vi "DOE Channel Test Labels.vi"(0 "RunTime":bool) -> (4 "Agilent Cluster Array":T2[](array[typedef]), 6 "Channel List":string)   [LabVIEW 2013]
uses:
  Type Definitions/Channel Label.ctl
  Type Definitions/Agilent Cluster.ctl
  <vilib>/Utility/file.llb/Write To Spreadsheet File (string).vi
  <vilib>/Utility/file.llb/Read From Spreadsheet File (string).vi
panel:
  in  "Sensor 5":T1
  in  "Read TC Tree":bool
  out "Description":string="DAQ Setup"
  in  "Tab Control":enum32{"Page 1", "Page 2"}(tab)
  out "Agilent TC Locations":string[][](array[string])
  in  "Read":bool
  in  "Write":bool
  in  "Sensor 4":T1
  in  "Read None":bool
  in  "Sensor 3":T1
  in  "Read All":bool
  in  "Complete":bool
  in  "Panel 3":T1[][](array[typedef])=[[{"Label"="TC Cond1 - IN", "Chan"="301", "Rec"=TRUE, "Unit"=""}, {"Label"="TC Cond2", "Chan"="302", "Rec"=TRUE, "Unit"=""}, {"Label"="TC Cond3", "Chan"="303", "Rec"=TRUE, "Unit"=""}, {"Label"="TC Cond4", "Chan"="304", "Rec"=TRUE, "Unit"=""}, {"Label"="TC Cond5", "Chan"="305", "Rec"=TRUE, "Unit"=""}, {"Label"="TC Cond6", "Chan"="306", "Rec"=TRUE, "Unit"=""}], [{"Label"="TC Cond7", "Chan"="307", "Rec"=TRUE, "Unit"=""}, {"Label"="TC Cond8", "Chan"="308", "Rec"=TRUE, "Unit"=""}, {"Label"="TC Cond9", "Chan"="309", "Rec"=TRUE, "Unit"=""}, {"Label"="TC Cond10", "Chan"="310", "Rec"=TRUE, "Unit"=""}, {"Label"="TC Cond11", "Chan"="311", "Rec"=TRUE, "Unit"=""}, {"Label"="TC Cond12 - OUT", "Chan"="312", "Rec"=TRUE, "Unit"=""}], [{"Label"="TC Xtra 4", "Chan"="313", "Rec"=TRUE, "Unit"=""}, {"Label"="TC Xtra 5", "Chan"="314", "Rec"=TRUE, "Unit"=""}, {"Label"="TC Xtra 6", "Chan"="315", "Rec"=TRUE, "Unit"=""}, {"Label"="TC Xtra 7", "Chan"="316", "Rec"=TRUE, "Unit"=""}, {"Label"="TC Xtra 8", "Chan"="105", "Rec"=TRUE, "Unit"=""}, {"Label"="TC Xtra 9", "Chan"="106", "Rec"=TRUE, "Unit"=""}]]
  in  "Panel 2":T1[][](array[typedef])=[[{"Label"="TC Dry/W bulb 1", "Chan"="201", "Rec"=TRUE, "Unit"=""}, {"Label"="TC Dry/W bulb 2", "Chan"="202", "Rec"=TRUE, "Unit"=""}, {"Label"="TC Dry/W bulb 3", "Chan"="203", "Rec"=TRUE, "Unit"=""}, {"Label"="TC Dry/W bulb 4", "Chan"="204", "Rec"=TRUE, "Unit"=""}, {"Label"="TC Tsuction", "Chan"="205", "Rec"=TRUE, "Unit"=""}, {"Label"="TC Tdis", "Chan"="206", "Rec"=TRUE, "Unit"=""}], [{"Label"="TC Tret", "Chan"="207", "Rec"=TRUE, "Unit"=""}, {"Label"="TC Controls 1", "Chan"="208", "Rec"=TRUE, "Unit"=""}, {"Label"="TC Controls 2", "Chan"="209", "Rec"=TRUE, "Unit"=""}, {"Label"="TC Controls 3", "Chan"="210", "Rec"=TRUE, "Unit"=""}, {"Label"="TC Controls 4", "Chan"="211", "Rec"=TRUE, "Unit"=""}, {"Label"="TC Controls 5", "Chan"="212", "Rec"=TRUE, "Unit"=""}], [{"Label"="TC Shadow T1", "Chan"="213", "Rec"=TRUE, "Unit"=""}, {"Label"="TC Shadow T2", "Chan"="214", "Rec"=TRUE, "Unit"=""}, {"Label"="TC Shadow T3", "Chan"="215", "Rec"=TRUE, "Unit"=""}, {"Label"="TC Shadow T4", "Chan"="216", "Rec"=TRUE, "Unit"=""}, {"Label"="TC Shadow T5", "Chan"="107", "Rec"=TRUE, "Unit"=""}, {"Label"="TC Shadow T6", "Chan"="108", "Rec"=TRUE, "Unit"=""}]]
  in  "Panel 1":T1[][](array[typedef])=[[{"Label"="TC Tree 1 - TOP", "Chan"="", "Rec"=TRUE, "Unit"=""}, {"Label"="TC Tree 2", "Chan"="", "Rec"=TRUE, "Unit"=""}, {"Label"="TC Tree 3", "Chan"="", "Rec"=TRUE, "Unit"=""}, {"Label"="TC Tree 4", "Chan"="", "Rec"=TRUE, "Unit"=""}, {"Label"="TC Tree 5", "Chan"="", "Rec"=TRUE, "Unit"=""}, {"Label"="TC Tree 6 - BOT", "Chan"="", "Rec"=TRUE, "Unit"=""}], [{"Label"="TC Shell 1", "Chan"="", "Rec"=TRUE, "Unit"=""}, {"Label"="TC Shell 2", "Chan"="", "Rec"=TRUE, "Unit"=""}, {"Label"="TC Shell 3", "Chan"="", "Rec"=TRUE, "Unit"=""}, {"Label"="TC Shell 4", "Chan"="", "Rec"=TRUE, "Unit"=""}, {"Label"="TC Evap1 - IN", "Chan"="111", "Rec"=TRUE, "Unit"=""}, {"Label"="TC Evap2", "Chan"="112", "Rec"=TRUE, "Unit"=""}], [{"Label"="TC Evap3", "Chan"="113", "Rec"=TRUE, "Unit"=""}, {"Label"="TC Evap4", "Chan"="114", "Rec"=TRUE, "Unit"=""}, {"Label"="TC Evap5 - OUT", "Chan"="115", "Rec"=TRUE, "Unit"=""}, {"Label"="TC Xtra 1", "Chan"="116", "Rec"=TRUE, "Unit"=""}, {"Label"="TC Xtra 2", "Chan"="109", "Rec"=TRUE, "Unit"=""}, {"Label"="TC Xtra 3", "Chan"="1100", "Rec"=TRUE, "Unit"=""}]]
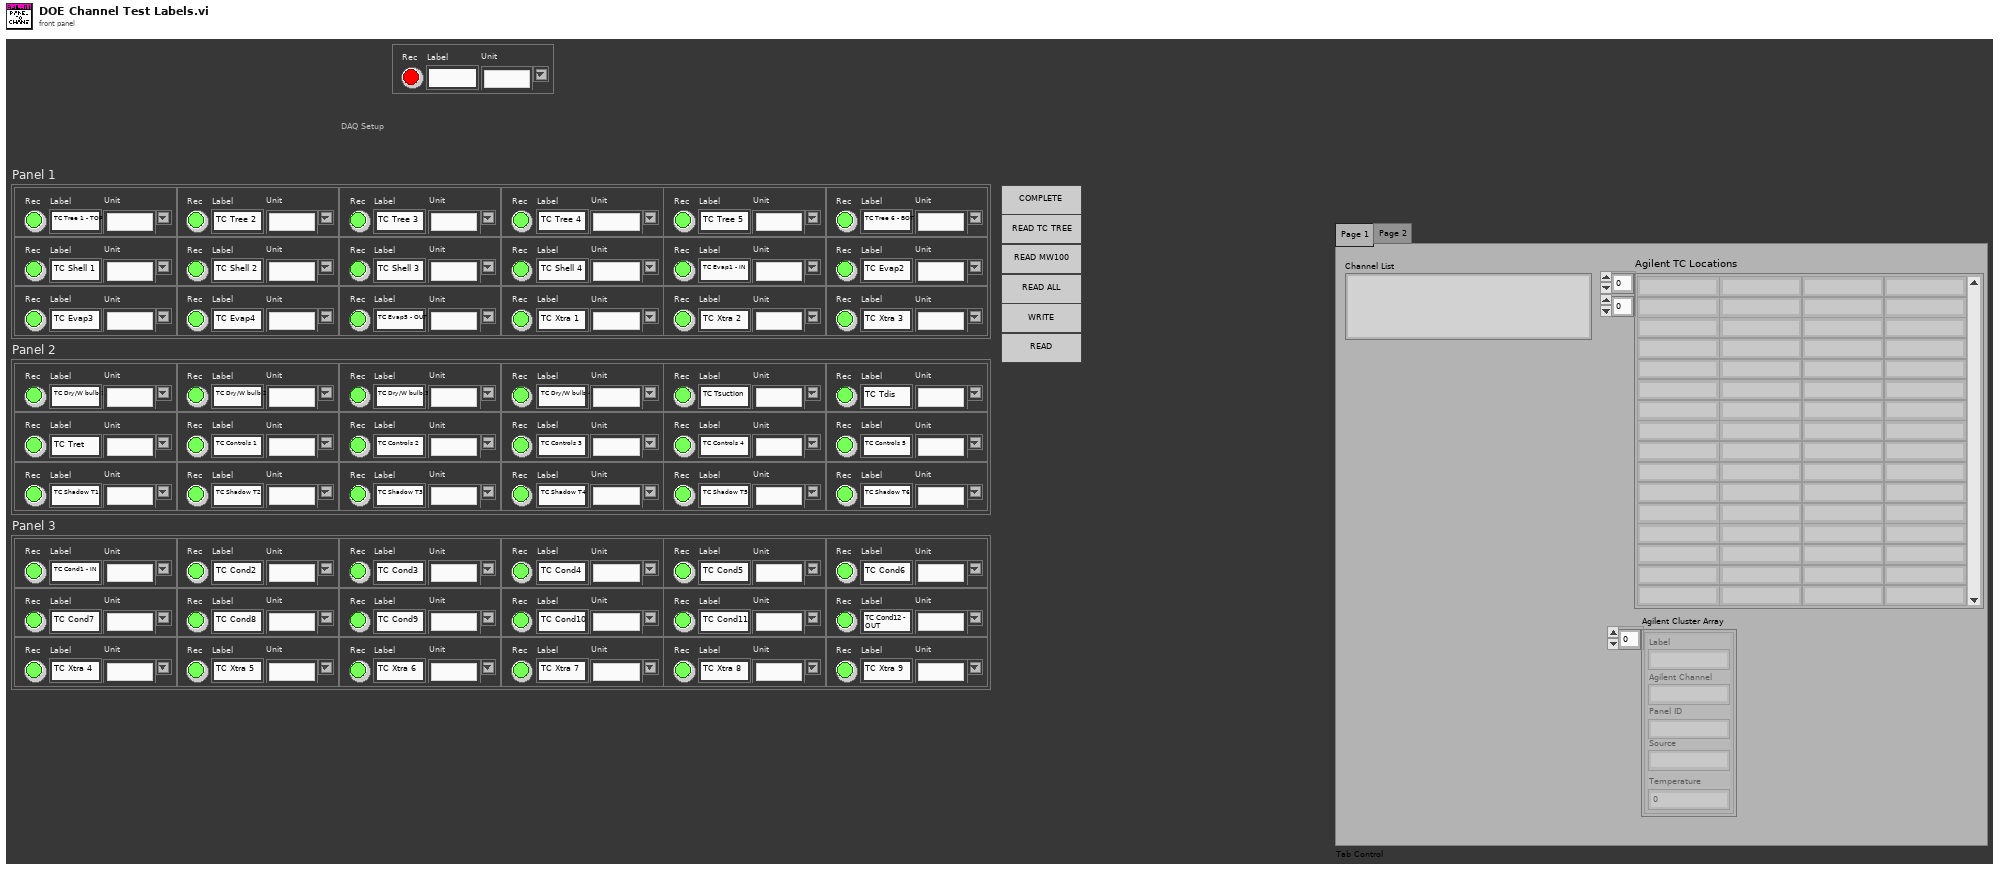
[diagram p1: front panel]
types:
  T1 = typedef "Channel Label.ctl" = cluster{"Label":string, "Chan":string, "Rec":bool, "Unit":string}
  T2 = typedef "Agilent Cluster.ctl" = cluster{"Label":string, "Agilent Channel":string, "Panel ID":string, "Source":string, "Temperature":dbl}
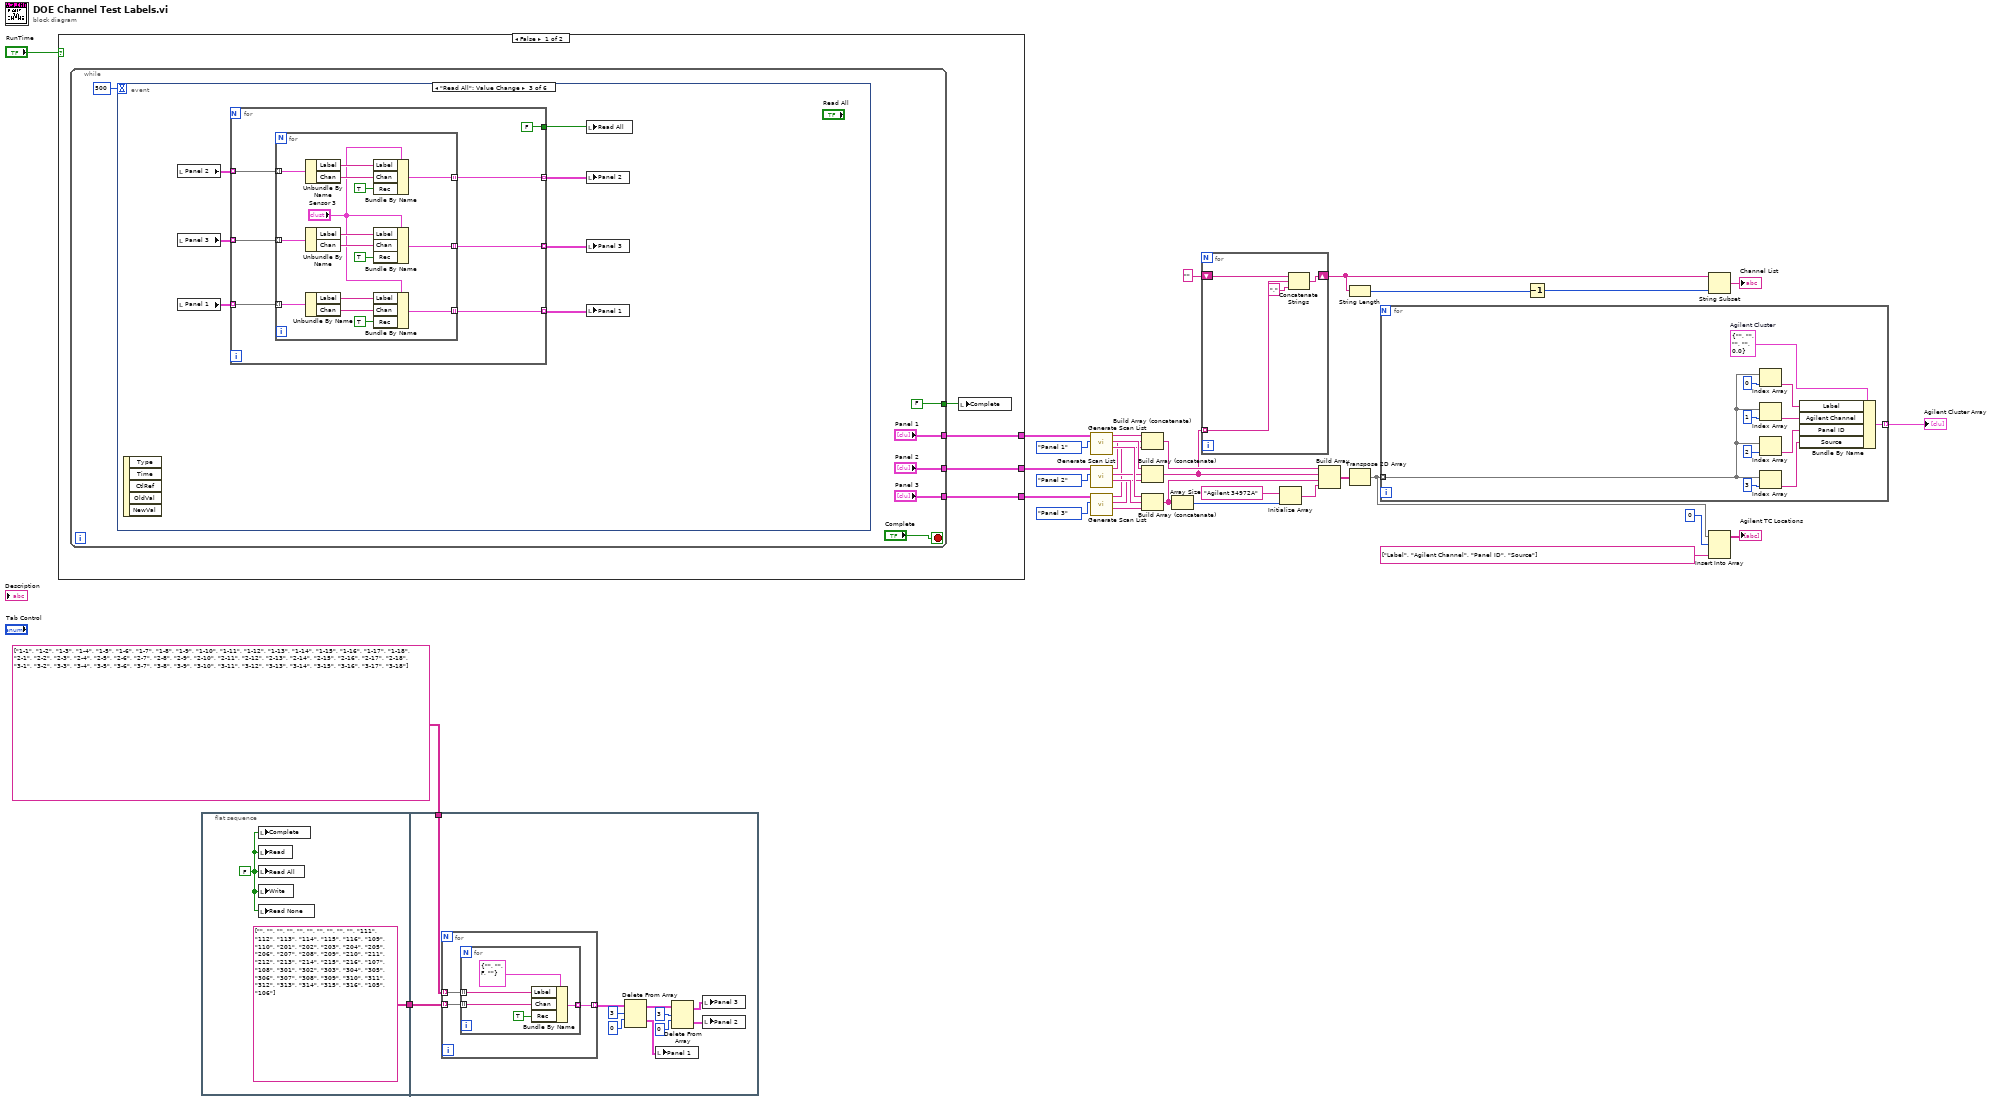
[diagram p0: block diagram]
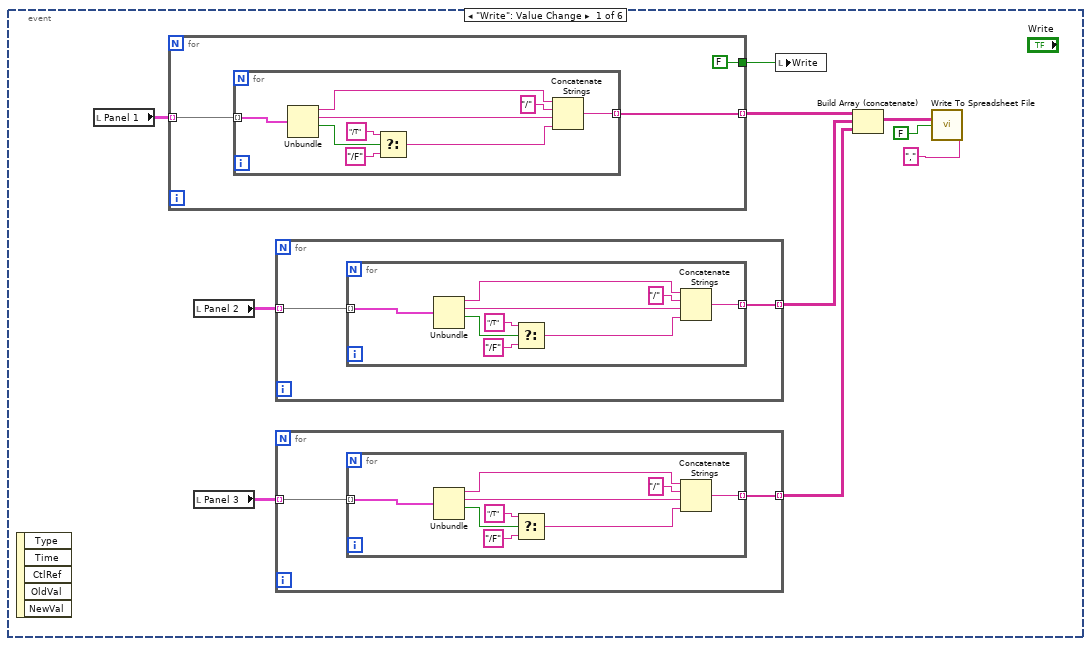
[diagram p2: hidden frame]
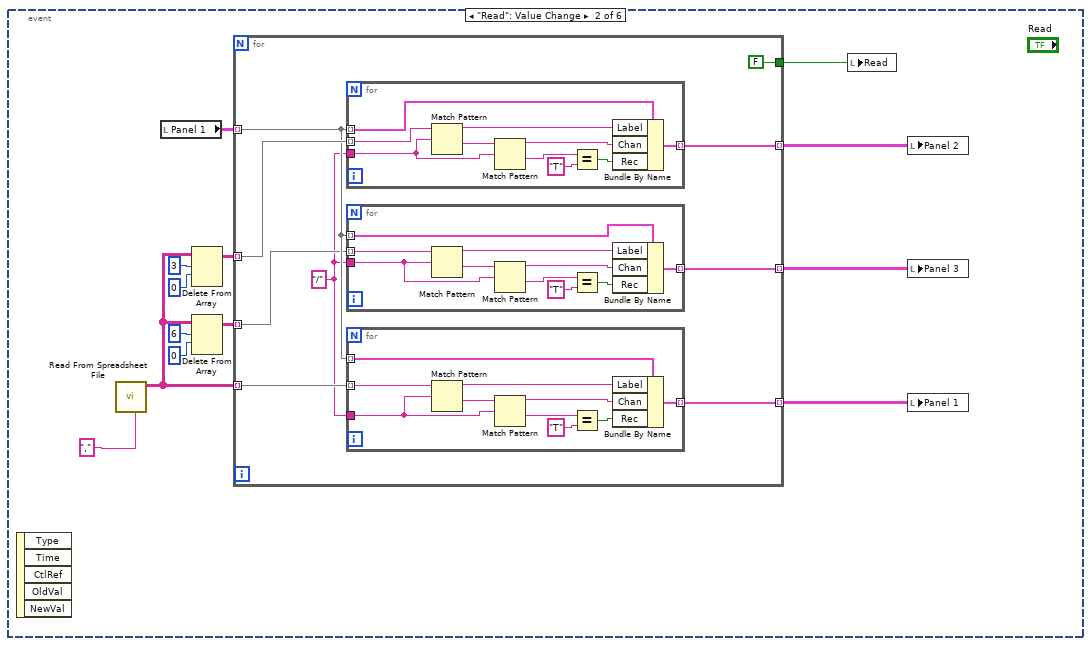
[diagram p3: hidden frame]
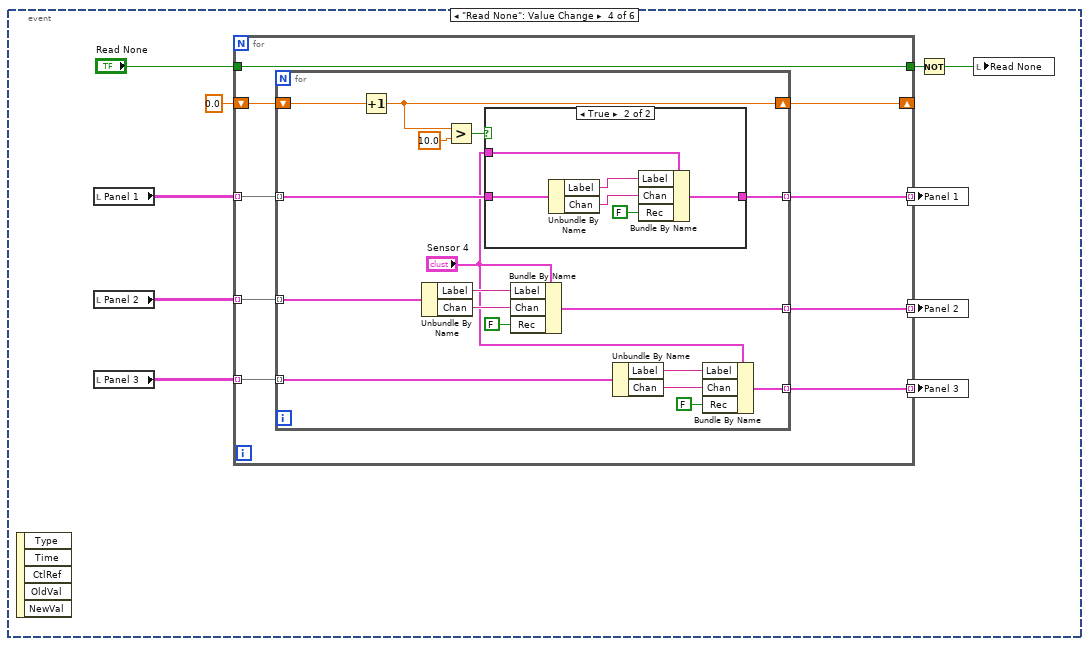
[diagram p4: hidden frame]
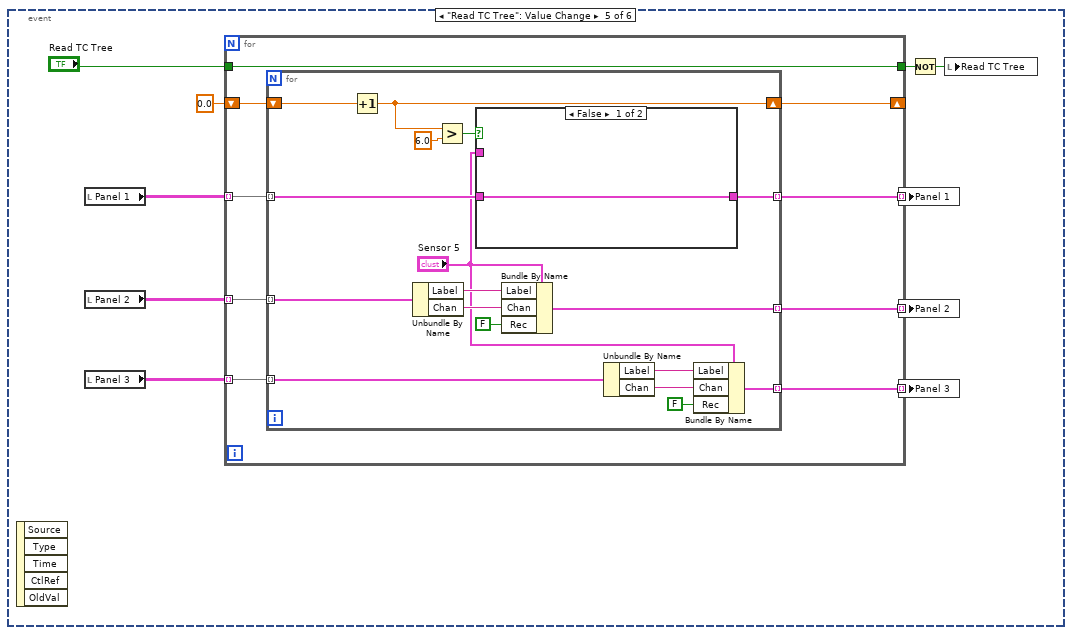
[diagram p6: hidden frame]
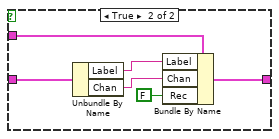
[diagram p7: hidden frame]
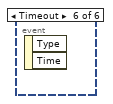
[diagram p8: hidden frame]
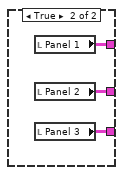
[diagram p9: hidden frame]
diagram:
  n1 = case shown="False" "RunTime" {
    tunnel: [w39 w260] -> w35
    tunnel: [w37 w259] -> w22
    tunnel: [w36 w258] -> w20
    frame False {
      n2 = while {
        tunnel: ["Panel 1"] -> w39
        tunnel: ["Panel 2"] -> w37
        tunnel: ["Panel 3"] -> w36
        tunnel: [FALSE ("Read None")] -> w38
        stop <- "Complete" stop-if-true
        n3 = event shown="[2] \"Read All\": Value Change" {
          selector: _ -> [_ _ _ _ _ _]
          dyn-events: _ -> [_ _ _ _ _ _]
          timeout: 500 -> [_ _ _ _ _ _]
          event "Write": Value Change {
            n4 = event-data() -> ()  [unwired: 1 in, 5 out]
            n5 = local read "Panel 1"() -> (w54:T1[][])
            n6 = for {
              tunnel: w54 -> [w80] mode=indexing
              tunnel: [FALSE ("Read None")] -> w55
              tunnel: [w78] -> w50 mode=indexing
              n7 = for {
                tunnel: w80 -> [w89] mode=indexing
                tunnel: [w81] -> w78 mode=indexing
                n8 = Unbundle(w89) -> ("Label"=w88:string, "Chan"=w86:string, "Rec"=w83:bool)  [unwired: 1 out]
                n9 = Select(t="/T" ("string"), s=w83, f="/F" ("string")) -> (s? t:f=w82:string)
                n10 = Concatenate Strings(w88, "/" ("string"), w86, w82) -> (w81:string)
              }
            }
            n11 = local read "Panel 2"() -> (w52:T1[][])
            n12 = local read "Panel 3"() -> (w51:T1[][])
            n13 = for {
              tunnel: w52 -> [w68] mode=indexing
              tunnel: [w67] -> w49 mode=indexing
              n14 = for {
                tunnel: w68 -> [w77] mode=indexing
                tunnel: [w69] -> w67 mode=indexing
                n15 = Unbundle(w77) -> ("Label"=w76:string, "Chan"=w74:string, "Rec"=w71:bool)  [unwired: 1 out]
                n16 = Select(t="/T" ("string"), s=w71, f="/F" ("string")) -> (s? t:f=w70:string)
                n17 = Concatenate Strings(w76, "/" ("string"), w74, w70) -> (w69:string)
              }
            }
            n18 = for {
              tunnel: w51 -> [w57] mode=indexing
              tunnel: [w56] -> w48 mode=indexing
              n19 = for {
                tunnel: w57 -> [w66] mode=indexing
                tunnel: [w58] -> w56 mode=indexing
                n20 = Unbundle(w66) -> ("Label"=w65:string, "Chan"=w63:string, "Rec"=w60:bool)  [unwired: 1 out]
                n21 = Select(t="/T" ("string"), s=w60, f="/F" ("string")) -> (s? t:f=w59:string)
                n22 = Concatenate Strings(w65, "/" ("string"), w63, w59) -> (w58:string)
              }
            }
            n23 = local write "Write"(w55) -> ()
            n24 = Build Array (concatenate)(w50, w49, w48) -> (w47:string[][])
            n25 = call-poly <vilib>:"Write To Spreadsheet File.vi"("2D data"=w47, "Keep Refnum Open"=FALSE, "delimiter (\\t)"="," ("delimiter (\\t)")) -> ()  [unwired: 11 in, 2 out]
          }
          event "Read": Value Change {
            n26 = event-data() -> ()  [unwired: 1 in, 5 out]
            n27 = call-poly <vilib>:"Read From Spreadsheet File.vi"("delimiter (\\t)"="," ("delimiter (\\t)")) -> ("all rows"=w96:string[][])  [unwired: 6 in, 4 out]
            n28 = local read "Panel 1"() -> (w92:T1[][])
            n29 = Delete From Array(array=w96, length=3, index (row)=0) -> (array with subset deleted=w97:string[][])  [unwired: 1 in, 1 out]
            n30 = Delete From Array(array=w96, length=6, index (row)=0) -> (array with subset deleted=w98:string[][])  [unwired: 1 in, 1 out]
            n31 = for {
              tunnel: w92 -> [w106] mode=indexing
              tunnel: w96 -> [w111] mode=indexing
              tunnel: [w110] -> w95 mode=indexing
              tunnel: w97 -> [w109] mode=indexing
              tunnel: w98 -> [w105] mode=indexing
              tunnel: [w108] -> w94 mode=indexing
              tunnel: [w107] -> w93 mode=indexing
              tunnel: [FALSE ("Read")] -> w91
              w104 = "/" ("regular expression")
              n32 = for {
                tunnel: w106 -> [w130] mode=indexing
                tunnel: w109 -> [w131] mode=indexing
                tunnel: [w128] -> w108 mode=indexing
                tunnel: w104 -> [w122]
                n33 = Match Pattern(string=w131, regular expression=w122) -> (before substring=w129:string, after substring=w127:string)  [unwired: 1 in, 2 out]
                n34 = Match Pattern(string=w127, regular expression=w122) -> (before substring=w126:string, after substring=w125:string)  [unwired: 1 in, 2 out]
                n35 = Equal?(x=w125, y="T") -> (x = y?=w123:bool)
                n36 = Bundle By Name(cluster=w130, "Label"=w129, "Chan"=w126, "Rec"=w123) -> (w128:T1)
              }
              n37 = for {
                tunnel: w106 -> [w120] mode=indexing
                tunnel: w105 -> [w121] mode=indexing
                tunnel: [w118] -> w107 mode=indexing
                tunnel: w104 -> [w112]
                n38 = Match Pattern(string=w121, regular expression=w112) -> (before substring=w119:string, after substring=w117:string)  [unwired: 1 in, 2 out]
                n39 = Match Pattern(string=w117, regular expression=w112) -> (before substring=w116:string, after substring=w115:string)  [unwired: 1 in, 2 out]
                n40 = Equal?(x=w115, y="T") -> (x = y?=w113:bool)
                n41 = Bundle By Name(cluster=w120, "Label"=w119, "Chan"=w116, "Rec"=w113) -> (w118:T1)
              }
              n42 = for {
                tunnel: w106 -> [w140] mode=indexing
                tunnel: w111 -> [w141] mode=indexing
                tunnel: [w138] -> w110 mode=indexing
                tunnel: w104 -> [w132]
                n43 = Match Pattern(string=w141, regular expression=w132) -> (before substring=w139:string, after substring=w137:string)  [unwired: 1 in, 2 out]
                n44 = Match Pattern(string=w137, regular expression=w132) -> (before substring=w136:string, after substring=w135:string)  [unwired: 1 in, 2 out]
                n45 = Equal?(x=w135, y="T") -> (x = y?=w133:bool)
                n46 = Bundle By Name(cluster=w140, "Label"=w139, "Chan"=w136, "Rec"=w133) -> (w138:T1)
              }
            }
            n47 = local write "Read"(w91) -> ()
            n48 = local write "Panel 2"(w94) -> ()
            n49 = local write "Panel 3"(w93) -> ()
            n50 = local write "Panel 1"(w95) -> ()
          }
          event "Read All": Value Change {
            n51 = event-data() -> ()  [unwired: 1 in, 5 out]
            n52 = local read "Panel 2"() -> (w145:T1[][])
            n53 = local read "Panel 3"() -> (w144:T1[][])
            n54 = local read "Panel 1"() -> (w148:T1[][])
            n55 = for {
              tunnel: [w155] -> w147 mode=indexing
              tunnel: w148 -> [w154] mode=indexing
              tunnel: [w153] -> w146 mode=indexing
              tunnel: w145 -> [w152] mode=indexing
              tunnel: w144 -> [w151] mode=indexing
              tunnel: [w150] -> w143 mode=indexing
              tunnel: [FALSE ("Read None")] -> w142
              n56 = for {
                tunnel: [w171] -> w155 mode=indexing
                tunnel: w154 -> [w169] mode=indexing
                tunnel: [w163] -> w153 mode=indexing
                tunnel: w152 -> [w162] mode=indexing
                tunnel: w151 -> [w158] mode=indexing
                tunnel: [w157] -> w150 mode=indexing
                n57 = Unbundle By Name(w162) -> ("Label"=w165:string, "Chan"=w166:string)
                n58 = Unbundle By Name(w158) -> ("Label"=w160:string, "Chan"=w159:string)
                n59 = Unbundle By Name(w169) -> ("Label"=w168:string, "Chan"=w167:string)
                n60 = Bundle By Name(cluster="Sensor 3", "Label"=w165, "Chan"=w166, "Rec"=TRUE) -> (w163:T1)
                n61 = Bundle By Name(cluster="Sensor 3", "Label"=w160, "Chan"=w159, "Rec"=TRUE) -> (w157:T1)
                n62 = Bundle By Name(cluster="Sensor 3", "Label"=w168, "Chan"=w167, "Rec"=TRUE) -> (w171:T1)
              }
            }
            n63 = local write "Read All"(w142) -> ()
            n64 = local write "Panel 2"(w146) -> ()
            n65 = local write "Panel 3"(w143) -> ()
            n66 = local write "Panel 1"(w147) -> ()
          }
          event "Read None": Value Change {
            n67 = event-data() -> ()  [unwired: 1 in, 5 out]
            n68 = local read "Panel 1"() -> (w181:T1[][])
            n69 = local read "Panel 2"() -> (w178:T1[][])
            n70 = local read "Panel 3"() -> (w177:T1[][])
            n71 = for {
              tunnel: [w190] -> w180 mode=indexing
              tunnel: w181 -> [w189] mode=indexing
              tunnel: [w188] -> w179 mode=indexing
              tunnel: w178 -> [w187] mode=indexing
              tunnel: w177 -> [w186] mode=indexing
              tunnel: [w185] -> w176 mode=indexing
              tunnel: [w184] -> w174
              tunnel: "Read None" -> [w184]
              shift-right: [w182] -> _
              shift-left: 0.0 -> [w183]
              n72 = for {
                tunnel: [w207] -> w190 mode=indexing
                tunnel: w189 -> [w206] mode=indexing
                tunnel: [w202] -> w188 mode=indexing
                tunnel: w187 -> [w201] mode=indexing
                tunnel: w186 -> [w197] mode=indexing
                tunnel: [w196] -> w185 mode=indexing
                shift-right: [w193] -> w182
                shift-left: w183 -> [w194]
                n73 = Increment(x=w194) -> (x+1=w193:dbl)
                n74 = Unbundle By Name(w201) -> ("Label"=w204:string, "Chan"=w205:string)
                n75 = Greater?(x=w193, y=10.0) -> (0:w191:bool)
                n76 = case shown="True" w191 {
                  tunnel: [w208 w214] -> w207
                  tunnel: w206 -> [w208 w212]
                  tunnel: "Sensor 4" -> [_ w209]
                  frame False {
                  }
                  frame True {
                    n77 = Unbundle By Name(w212) -> ("Label"=w211:string, "Chan"=w210:string)
                    n78 = Bundle By Name(cluster=w209, "Label"=w211, "Chan"=w210, "Rec"=FALSE) -> (w214:T1)
                  }
                }
                n79 = Bundle By Name(cluster="Sensor 4", "Label"=w204, "Chan"=w205, "Rec"=FALSE) -> (w202:T1)
                n80 = Unbundle By Name(w197) -> ("Label"=w199:string, "Chan"=w198:string)
                n81 = Bundle By Name(cluster="Sensor 4", "Label"=w199, "Chan"=w198, "Rec"=FALSE) -> (w196:T1)
              }
            }
            n82 = local write "Panel 1"(w180) -> ()
            n83 = local write "Panel 2"(w179) -> ()
            n84 = local write "Panel 3"(w176) -> ()
            n85 = Not(x=w174) -> (.not. x?=w175:bool)
            n86 = local write "Read None"(w175) -> ()
          }
          event "Read TC Tree": Value Change {
            n87 = event-data() -> ()  [unwired: 1 in, 5 out]
            n88 = local read "Panel 1"() -> (w224:T1[][])
            n89 = local read "Panel 2"() -> (w221:T1[][])
            n90 = local read "Panel 3"() -> (w220:T1[][])
            n91 = for {
              tunnel: [w233] -> w223 mode=indexing
              tunnel: w224 -> [w232] mode=indexing
              tunnel: [w231] -> w222 mode=indexing
              tunnel: w221 -> [w230] mode=indexing
              tunnel: w220 -> [w229] mode=indexing
              tunnel: [w228] -> w219 mode=indexing
              tunnel: [w227] -> w218
              tunnel: "Read TC Tree" -> [w227]
              shift-right: [w225] -> _
              shift-left: 0.0 -> [w226]
              n92 = for {
                tunnel: [w250] -> w233 mode=indexing
                tunnel: w232 -> [w249] mode=indexing
                tunnel: [w245] -> w231 mode=indexing
                tunnel: w230 -> [w244] mode=indexing
                tunnel: w229 -> [w240] mode=indexing
                tunnel: [w239] -> w228 mode=indexing
                shift-right: [w236] -> w225
                shift-left: w226 -> [w237]
                n93 = Increment(x=w237) -> (x+1=w236:dbl)
                n94 = Unbundle By Name(w244) -> ("Label"=w247:string, "Chan"=w248:string)
                n95 = Greater?(x=w236, y=6.0) -> (0:w234:bool)
                n96 = case shown="False" w234 {
                  tunnel: [w251 w257] -> w250
                  tunnel: w249 -> [w251 w255]
                  tunnel: "Sensor 5" -> [_ w252]
                  frame False {
                  }
                  frame True {
                    n97 = Unbundle By Name(w255) -> ("Label"=w254:string, "Chan"=w253:string)
                    n98 = Bundle By Name(cluster=w252, "Label"=w254, "Chan"=w253, "Rec"=FALSE) -> (w257:T1)
                  }
                }
                n99 = Bundle By Name(cluster="Sensor 5", "Label"=w247, "Chan"=w248, "Rec"=FALSE) -> (w245:T1)
                n100 = Unbundle By Name(w240) -> ("Label"=w242:string, "Chan"=w241:string)
                n101 = Bundle By Name(cluster="Sensor 5", "Label"=w242, "Chan"=w241, "Rec"=FALSE) -> (w239:T1)
              }
            }
            n102 = local write "Panel 1"(w223) -> ()
            n103 = local write "Panel 2"(w222) -> ()
            n104 = local write "Panel 3"(w219) -> ()
            n105 = Not(x=w218) -> (.not. x?=w215:bool)
            n106 = local write "Read TC Tree"(w215) -> ()
          }
          event Timeout {
            n107 = event-data() -> ()  [unwired: 1 in, 2 out]
          }
        }
      }
      n108 = local write "Complete"(w38) -> ()
    }
    frame True {
      n109 = local read "Panel 1"() -> (w260:T1[][])
      n110 = local read "Panel 2"() -> (w259:T1[][])
      n111 = local read "Panel 3"() -> (w258:T1[][])
    }
  }
  n112 = flat-sequence {
    tunnel: [string[][] [["", "", "", "", "", ""], ["", "", "", "", "111", "112"], ["113", "114", "115", "116", "109", "110"], ["201", "202", "203", "204", "205", "206"], ["207", "208", "209", "210", "211", "212"], ["213", "214", "215", "216", "107", "108"], ["301", "302", "303", "304", "305", "306"], ["307", "308", "309", "310", "311", "312"], ["313", "314", "315", "316", "105", "106"]] ("transposed array")] -> w12
    tunnel: w12 -> [w264]
    tunnel: string[][] [["1-1", "1-2", "1-3", "1-4", "1-5", "1-6"], ["1-7", "1-8", "1-9", "1-10", "1-11", "1-12"], ["1-13", "1-14", "1-15", "1-16", "1-17", "1-18"], ["2-1", "2-2", "2-3", "2-4", "2-5", "2-6"], ["2-7", "2-8", "2-9", "2-10", "2-11", "2-12"], ["2-13", "2-14", "2-15", "2-16", "2-17", "2-18"], ["3-1", "3-2", "3-3", "3-4", "3-5", "3-6"], ["3-7", "3-8", "3-9", "3-10", "3-11", "3-12"], ["3-13", "3-14", "3-15", "3-16", "3-17", "3-18"]] ("Array") -> [w263]
    frame #0 {
      w261 = FALSE ("Read None")
      n113 = local write "Complete"(w261) -> ()
      n114 = local write "Read"(w261) -> ()
      n115 = local write "Read All"(w261) -> ()
      n116 = local write "Write"(w261) -> ()
      n117 = local write "Read None"(w261) -> ()
    }
    frame #1 {
      n118 = for {
        tunnel: [w276] -> w273 mode=indexing
        tunnel: w263 -> [w275] mode=indexing
        tunnel: w264 -> [w274] mode=indexing
        n119 = for {
          tunnel: [w281] -> w276 mode=indexing
          tunnel: w275 -> [w280] mode=indexing
          tunnel: w274 -> [w279] mode=indexing
          n120 = Bundle By Name(cluster=T1 {"Label"="", "Chan"="", "Rec"=FALSE, "Unit"=""} ("Sensor 2"), "Label"=w280, "Chan"=w279, "Rec"=TRUE) -> (w281:T1)
        }
      }
      n121 = Delete From Array(array=w273, length=3, index (row)=0) -> (deleted portion=w267:T1[][], array with subset deleted=w268:T1[][])  [unwired: 1 in]
      n122 = local write "Panel 1"(w267) -> ()
      n123 = Delete From Array(array=w268, length=3, index (row)=0) -> (deleted portion=w266:T1[][], array with subset deleted=w265:T1[][])  [unwired: 1 in]
      n124 = local write "Panel 3"(w265) -> ()
      n125 = local write "Panel 2"(w266) -> ()
    }
  }
  n126 = call "Generate Scan List.vi"(10:"Panel"=enum16{"Panel 1", "Panel 2", "Panel 3"}."Panel 1" ("Panel"), 11:"Panel"=w35) -> ("Panel List"=w27:string[], "Channel Number"=w33:string[], "Channel Label"=w34:string[])  [unwired: 7 in]
  n127 = call "Generate Scan List.vi"(10:"Panel"=enum16{"Panel 1", "Panel 2", "Panel 3"}."Panel 2" ("Panel"), 11:"Panel"=w22) -> ("Panel List"=w18:string[], "Channel Number"=w16:string[], "Channel Label"=w17:string[])  [unwired: 7 in]
  n128 = call "Generate Scan List.vi"(10:"Panel"=enum16{"Panel 1", "Panel 2", "Panel 3"}."Panel 3" ("Panel"), 11:"Panel"=w20) -> ("Panel List"=w15:string[], "Channel Number"=w13:string[], "Channel Label"=w14:string[])  [unwired: 7 in]
  n129 = Build Array (concatenate)(w34, w17, w14) -> (w26:string[])
  n130 = Build Array (concatenate)(w33, w16, w13) -> (w25:string[])
  n131 = Build Array (concatenate)(w27, w18, w15) -> (w5:string[])
  n132 = Array Size(array=w5) -> (size(s)=w4:i32)
  n133 = for {
    tunnel: w25 -> [w284] mode=indexing
    shift-right: [w283] -> w31
    shift-left: "" -> [w282]
    n134 = Concatenate Strings(w282, w284, "," ("string")) -> (w283:string)
  }
  n135 = Initialize Array("Agilent 34972A", w4) -> (w3:string[])
  n136 = Build Array(w26, w25, w5, w3) -> (w24:string[][])
  n137 = String Length(string=w31) -> (length=w29:i32)
  n138 = Transpose 2D Array(2D array=w24) -> (transposed array=w2:string[][])
  n139 = for {
    tunnel: w2 -> [w296] mode=indexing
    tunnel: [w287] -> w1 mode=indexing
    w286 = T2 {"Label"="", "Agilent Channel"="", "Panel ID"="", "Source"="", "Temperature"=0.0}  # Agilent Cluster
    n140 = Index Array(array=w296, index=0) -> (element=w291:string)
    n141 = Index Array(array=w296, index=1) -> (element=w290:string)
    n142 = Index Array(array=w296, index=2) -> (element=w289:string)
    n143 = Index Array(array=w296, index=3) -> (element=w288:string)
    n144 = Bundle By Name(cluster=w286, "Label"=w291, "Agilent Channel"=w290, "Panel ID"=w289, "Source"=w288) -> (w287:T2)
  }
  "Agilent Cluster Array" <- w1
  n145 = Decrement(x=w29) -> (x-1=w30:i32)
  n146 = String Subset(string=w31, length (rest)=w30) -> (substring=→"Channel List":string)  [unwired: 1 in]
  n147 = Insert Into Array(array=w2, index (row)=0, new element=string[] ["Label", "Agilent Channel", "Panel ID", "Source"] ("element")) -> (→"Agilent TC Locations":string[][])  [unwired: 1 in]
